vi "danteSendReceive_p.vi"() -> ()   [LabVIEW 2010]
uses:
  <vilib>/Utility/error.llb/DialogType.ctl
  <userlib>/libcommon_serial/libcommon_serial.lvlib
panel:
  out "QueryErrorDesc":string
  out "ReadErrorSpec":i32
  out "WriteErrorSpec":i32
  out "WriteErrorDesc":string
  out "ReadErrorDesc":string
  out "query sent":string
  out "QueryError":bool
  out "errorQuery":cdb format="%.2f"
  out "Error Testing Query":bool
  out "query return":string
  out "Byte received":i32[](array[numeric])
  out "Error testing ramp":bool
  in  "timeOut [ms] (1000)":i32=1000
  out "error Configuring":cdb format="%.2f"
  in  "subID2 (0)":u32
  in  "serialBoard":u16(ring) items=["ttyr", "ttyS"]
  out "Byte Sent":i32[](array[numeric])
  in  "Test Buffer size":i32=128
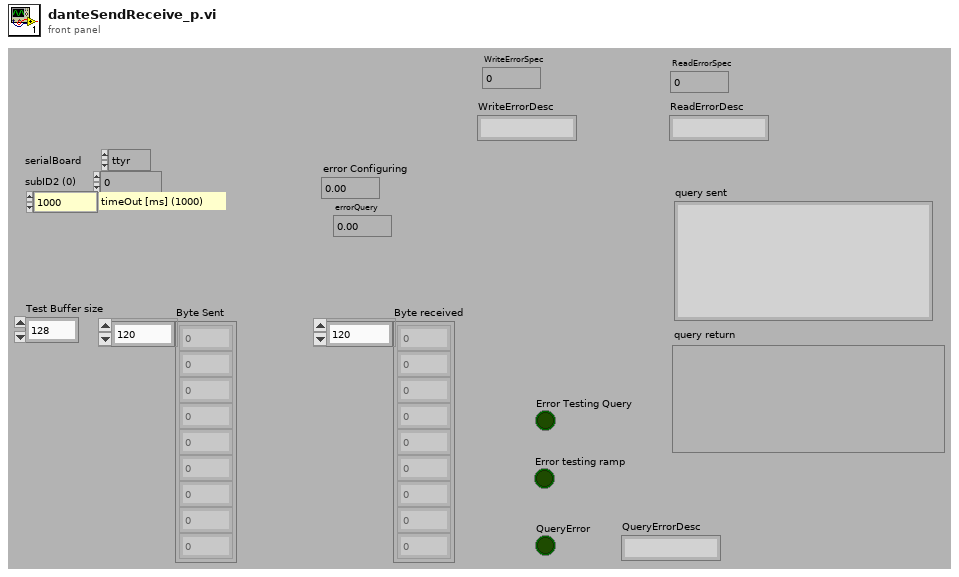
[diagram p1: front panel]
types:
  T1 = typedef "DialogType.ctl" = u16
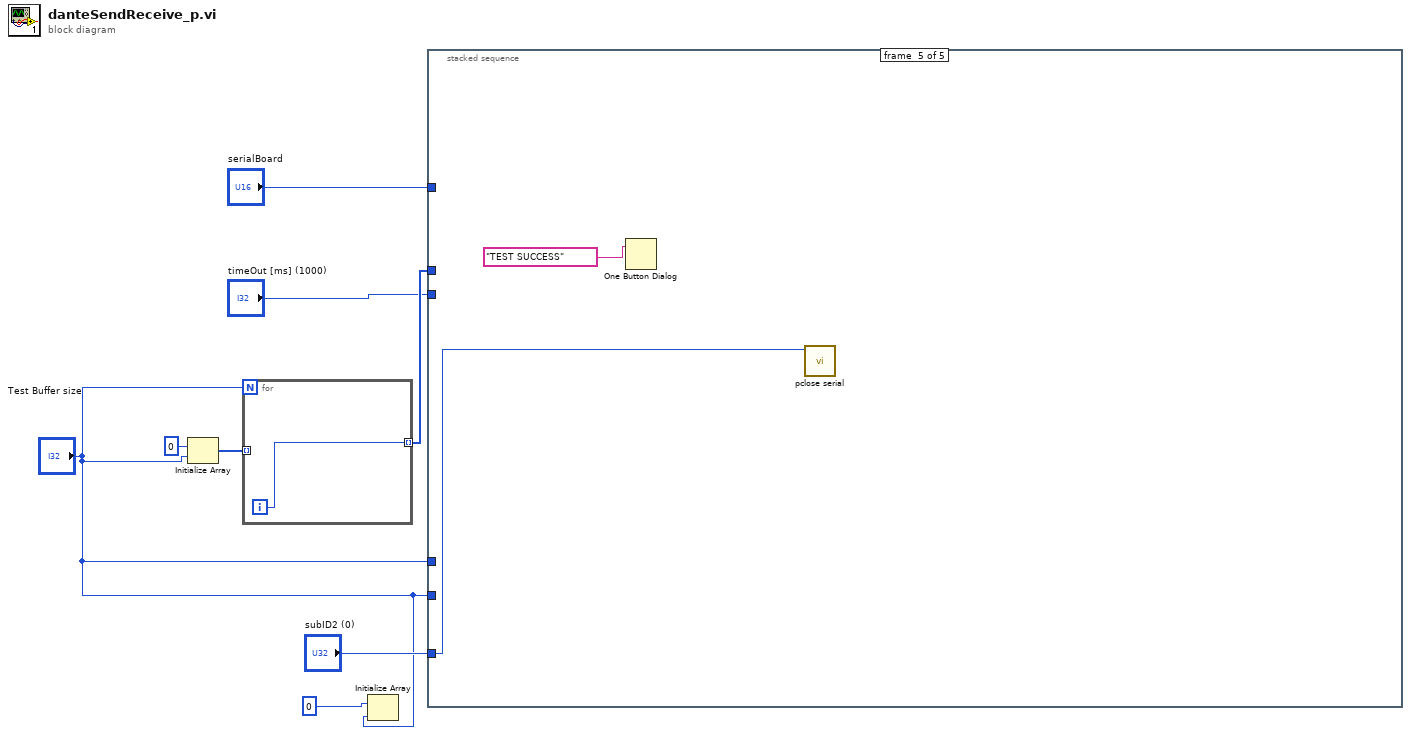
[diagram p0: block diagram]
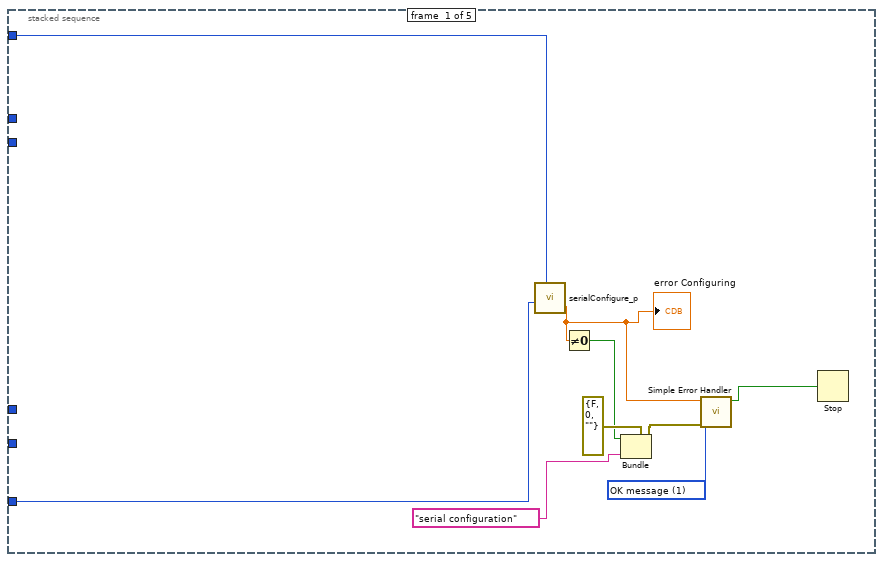
[diagram p2: hidden frame]
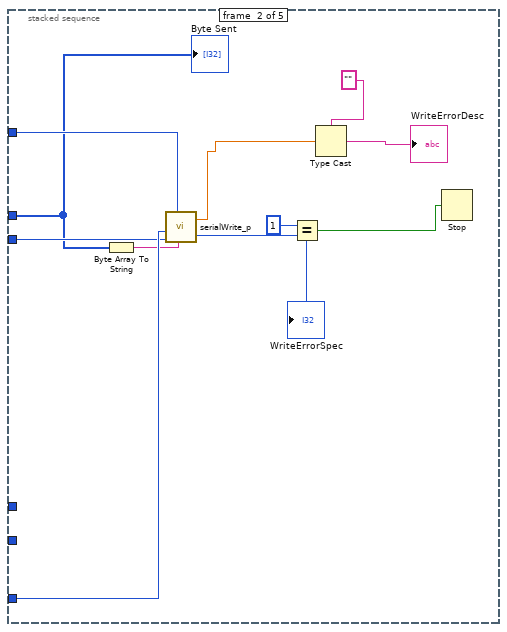
[diagram p3: hidden frame]
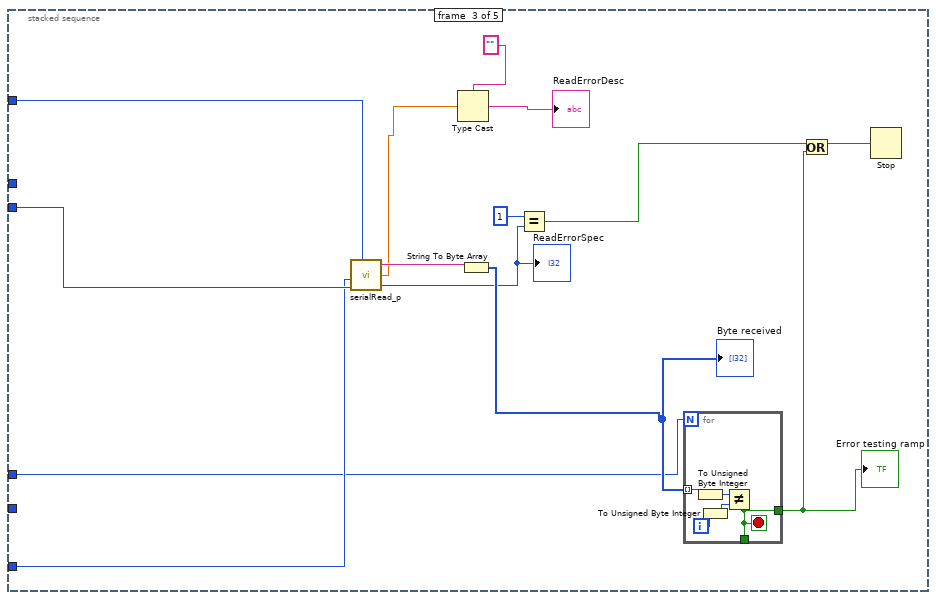
[diagram p4: hidden frame]
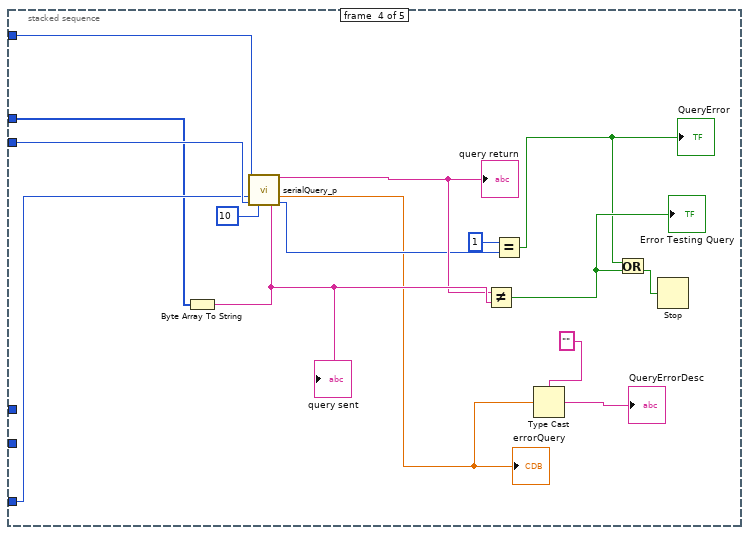
[diagram p5: hidden frame]
diagram:
  n1 = Initialize Array(i8 0 ("element"), "Test Buffer size") -> (w7:i8[])
  n2 = for {
    N: "Test Buffer size" -> [_]
    tunnel: w7 -> [_] mode=indexing
    tunnel: [w9] -> w6 mode=indexing
    i -> [w9]
  }
  n3 = Initialize Array(i8 0 ("element"), "Test Buffer size") -> ()  [unwired: 1 out]
  n4 = stacked-sequence {
    tunnel: w6 -> [_ w26 _ w59 _]
    tunnel: "Test Buffer size" -> [_ _ _ _ _]
    tunnel: "serialBoard" -> [w16 w29 w41 w61 _]
    tunnel: "subID2 (0)" -> [w15 w28 w42 w62 w65]
    tunnel: "timeOut [ms] (1000)" -> [_ w27 w43 w63 _]
    tunnel: "Test Buffer size" -> [_ _ w30 _ _]
    frame #0 {
      w13 = T1 1 items=["no dialog", "OK message", "continue or stop message", "OK message + warnings", "continue/stop + warnings"] ("type of dialog (OK msg:1)")
      n5 = call "serialConfigure_p.vi"("serialBoard"=w16, "subID2 (0)"=w15) -> ("errorCode"=w12:cdb)  [unwired: 5 in]
      "error Configuring" <- w12
      n6 = Not Equal To 0?(x=w12) -> (x != 0?=w14:bool)
      n7 = Bundle(cluster=errorcluster {"status"=FALSE, "code"=0, "source"=""} ("error in (no error)"), "status"=w14, "source"="serial configuration" ("error source (\" \")")) -> (w17:errorcluster)  [unwired: 1 in]
      n8 = call <vilib>:"Simple Error Handler.vi"("error code (no error:0)"=w12, "type of dialog (OK msg:1)"=w13, "error in (no error)"=w17) -> ("error?"=w11:bool)  [unwired: 2 in, 4 out]
      n9 = Stop(stop? (T)=w11) -> ()
    }
    frame #1 {
      n10 = Byte Array To String(unsigned byte array=w26) -> (string=w25:string)
      n11 = call "serialWrite_p.vi"("string to write"=w25, "serialBoard"=w29, "timeOut [ms] (1000)"=w27, "subID2 (0)"=w28) -> ("errorSpec"=w20:i32, "errorCode"=w21:cdb)  [unwired: 2 in]
      "WriteErrorSpec" <- w20
      n12 = Equal?(x=1, y=w20) -> (x = y?=w24:bool)
      n13 = Type Cast(type="", x=w21) -> (*(type *) &x=→"WriteErrorDesc":string)
      n14 = Stop(stop? (T)=w24) -> ()
      "Byte Sent" <- w26
    }
    frame #2 {
      n15 = call "serialRead_p.vi"("serialBoard"=w41, "subID2 (0)"=w42, "timeOut [ms] (1000)"=w43) -> ("string read"=w40:string, "errorCode"=w34:cdb, "errorSpec"=w37:i32)  [unwired: 3 in]
      "ReadErrorSpec" <- w37
      n16 = Type Cast(type="", x=w34) -> (*(type *) &x=→"ReadErrorDesc":string)
      n17 = String To Byte Array(string=w40) -> (unsigned byte array=w39:u8[])
      "Byte received" <- w39
      n18 = Equal?(x=1, y=w37) -> (x = y?=w38:bool)
      n19 = for {
        N: w30 -> [_]
        tunnel: w39 -> [w47] mode=indexing
        tunnel: [w44] -> _
        tunnel: [w44] -> w31
        i -> [w48]
        stop <- w44 stop-if-true
        n20 = To Unsigned Byte Integer(number=w47) -> (unsigned 8bit integer=w46:u8)
        n21 = To Unsigned Byte Integer(number=w48) -> (unsigned 8bit integer=w45:u8)
        n22 = Not Equal?(x=w46, y=w45) -> (x != y?=w44:bool)
      }
      "Error testing ramp" <- w31
      n23 = Or(x=w38, y=w31) -> (x .or. y?=w32:bool)
      n24 = Stop(stop? (T)=w32) -> ()
    }
    frame #3 {
      n25 = Byte Array To String(unsigned byte array=w59) -> (string=w58:string)
      "query sent" <- w58
      n26 = call "serialQuery_p.vi"("serialBoard"=w61, "subID2 (0)"=w62, "timeOut [ms] (1000)"=w63, "wait [ms] (1000)"=10, "string to write"=w58) -> ("string read"=w57:string, "errorCode"=w52:cdb, "errorSpec"=w56:i32)  [unwired: 8 in]
      "query return" <- w57
      "errorQuery" <- w52
      n27 = Not Equal?(x=w57, y=w58) -> (x != y?=w51:bool)
      "Error Testing Query" <- w51
      n28 = Equal?(x=1, y=w56) -> (x = y?=w49:bool)
      "QueryError" <- w49
      n29 = Type Cast(type="", x=w52) -> (*(type *) &x=→"QueryErrorDesc":string)
      n30 = Or(x=w49, y=w51) -> (x .or. y?=w50:bool)
      n31 = Stop(stop? (T)=w50) -> ()
    }
    frame #4 {
      n32 = One Button Dialog(message="TEST SUCCESS") -> ()  [unwired: 1 in, 1 out]
      n33 = call <userlib>:"pclose serial.vi"("resourceId"=w65) -> ()  [unwired: 9 in, 2 out]
    }
  }
